vi "RT_Transmission.vi"() -> ()   [LabVIEW 2016]
uses:
  <vilib>/Instr/_visa.llb/VISA Configure Serial Port (Instr).vi
  <vilib>/FPGAPlugInAG/cRIO-9067/niLvFpga_Open_cRIO-9067.vi
  <vilib>/Utility/error.llb/Error Cluster From Error Code.vi
  <vilib>/rvi/errors/niLvFpgaAdjustHostInterfaceError.vi
  <vilib>/functionblocks/Control/PID/PID.vi
  <vilib>/rvi/interface/nirviOpenFPGA/nirviOpenFPGA.xnode
  FPGA Bitfiles/MayUpgrade_FPGA-Trans_Transmission-FPG_MZXtHOBdRVI.lvbitx
  FPGA_Transmission.vi
  <vilib>/rvi/interface/nirviReadWriteControl/nirviReadWriteControl.xnode
  <vilib>/functionblocks/FB Core/FB Core.xnode
  <vilib>/functionblocks/NI_FunctionBlock Libraries.lvlib
  NiFpgaLv.dll
  <vilib>/rvi/errors/niLvFpgaMergeErrorWithErrorCode.vi
panel:
  in  "Tab Control":enum32{"control", "Junk"}(tab)
  out "Steerer X+":dbl
  out "Steerer X-":dbl
  out "Steerer Y+":dbl
  out "Steerer Y-":dbl
  out "ExB +":dbl
  out "ExB -":dbl
  out "X+ V":fxp<+/-,26,5> format="%.23g"
  out "X+ I":fxp<+/-,26,5> format="%_4g"
  out "X- V":fxp<+/-,26,5> format="%_4g"
  out "X-I":fxp<+/-,26,5> format="%_4g"
  out "Y+ V":fxp<+/-,26,5> format="%_4g"
  out "Y+I":fxp<+/-,26,5> format="%_4g"
  out "Y-V":fxp<+/-,26,5> format="%_4g"
  out "Y-I":fxp<+/-,26,5> format="%_4g"
  out "ExB + V":fxp<+/-,26,5> format="%_4g"
  out "ExB +I":fxp<+/-,26,5> format="%_4g"
  out "ExB -V":fxp<+/-,26,5> format="%_4g"
  out "ExB-I":fxp<+/-,26,5> format="%_4g"
  out "ExB Magnet command string":string
  out "Ion gauge switch object cluser 2":T1
  out "Ion gauge anal waist Cluster 1":T1
  out "EXB":dbl
  in  "derivative time (Td, min)":dbl=0.05
  in  "integral time (Ti, min)":dbl=0.01
  in  "proportional gain (Kc)":dbl=25.0
  out "Analyze Magnet command string":string
  out "anal field read":dbl
  out "unsigned byte array":u8[](array[numeric])
  out "Analyze read":u8[](array[numeric])
  out "analyze magnet set field":dbl
  out "element":dbl
  in  "diverter":bool
  out "diverter":bool
  out "ExB Magnet read string":string
  out "ExB Magnet read":dbl
  out "ExB loop error":errorcluster
  out "Analog control error":errorcluster
  out "FPGA error":errorcluster
  in  "Ion gauge cluster control":T1
  out "Convectron 3":u8[](array[numeric])
  out "Ion gauge 4":u8[](array[numeric])
  out "Convectron 4":u8[](array[numeric])
  out "Ion gauge 5":u8[](array[numeric])
  out "Convectron 2":u8[](array[numeric])
  out "Ion gauge 2":u8[](array[numeric])
  out "Convectron 1":u8[](array[numeric])
  out "Ion gauge 1":u8[](array[numeric])
  out "Vac Cluster Error":errorcluster
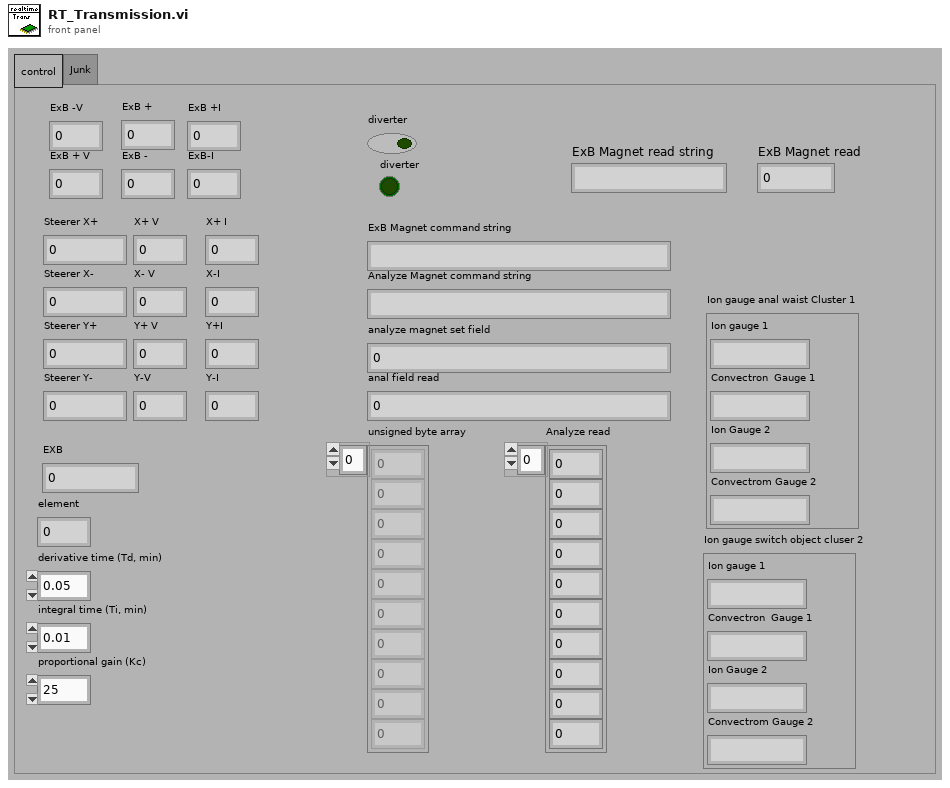
[diagram p1: front panel]
types:
  T1 = cluster{"Ion gauge 1":string, "Convectron  Gauge 1 ":string, "Ion Gauge 2":string, "Convectrom Gauge 2":string}
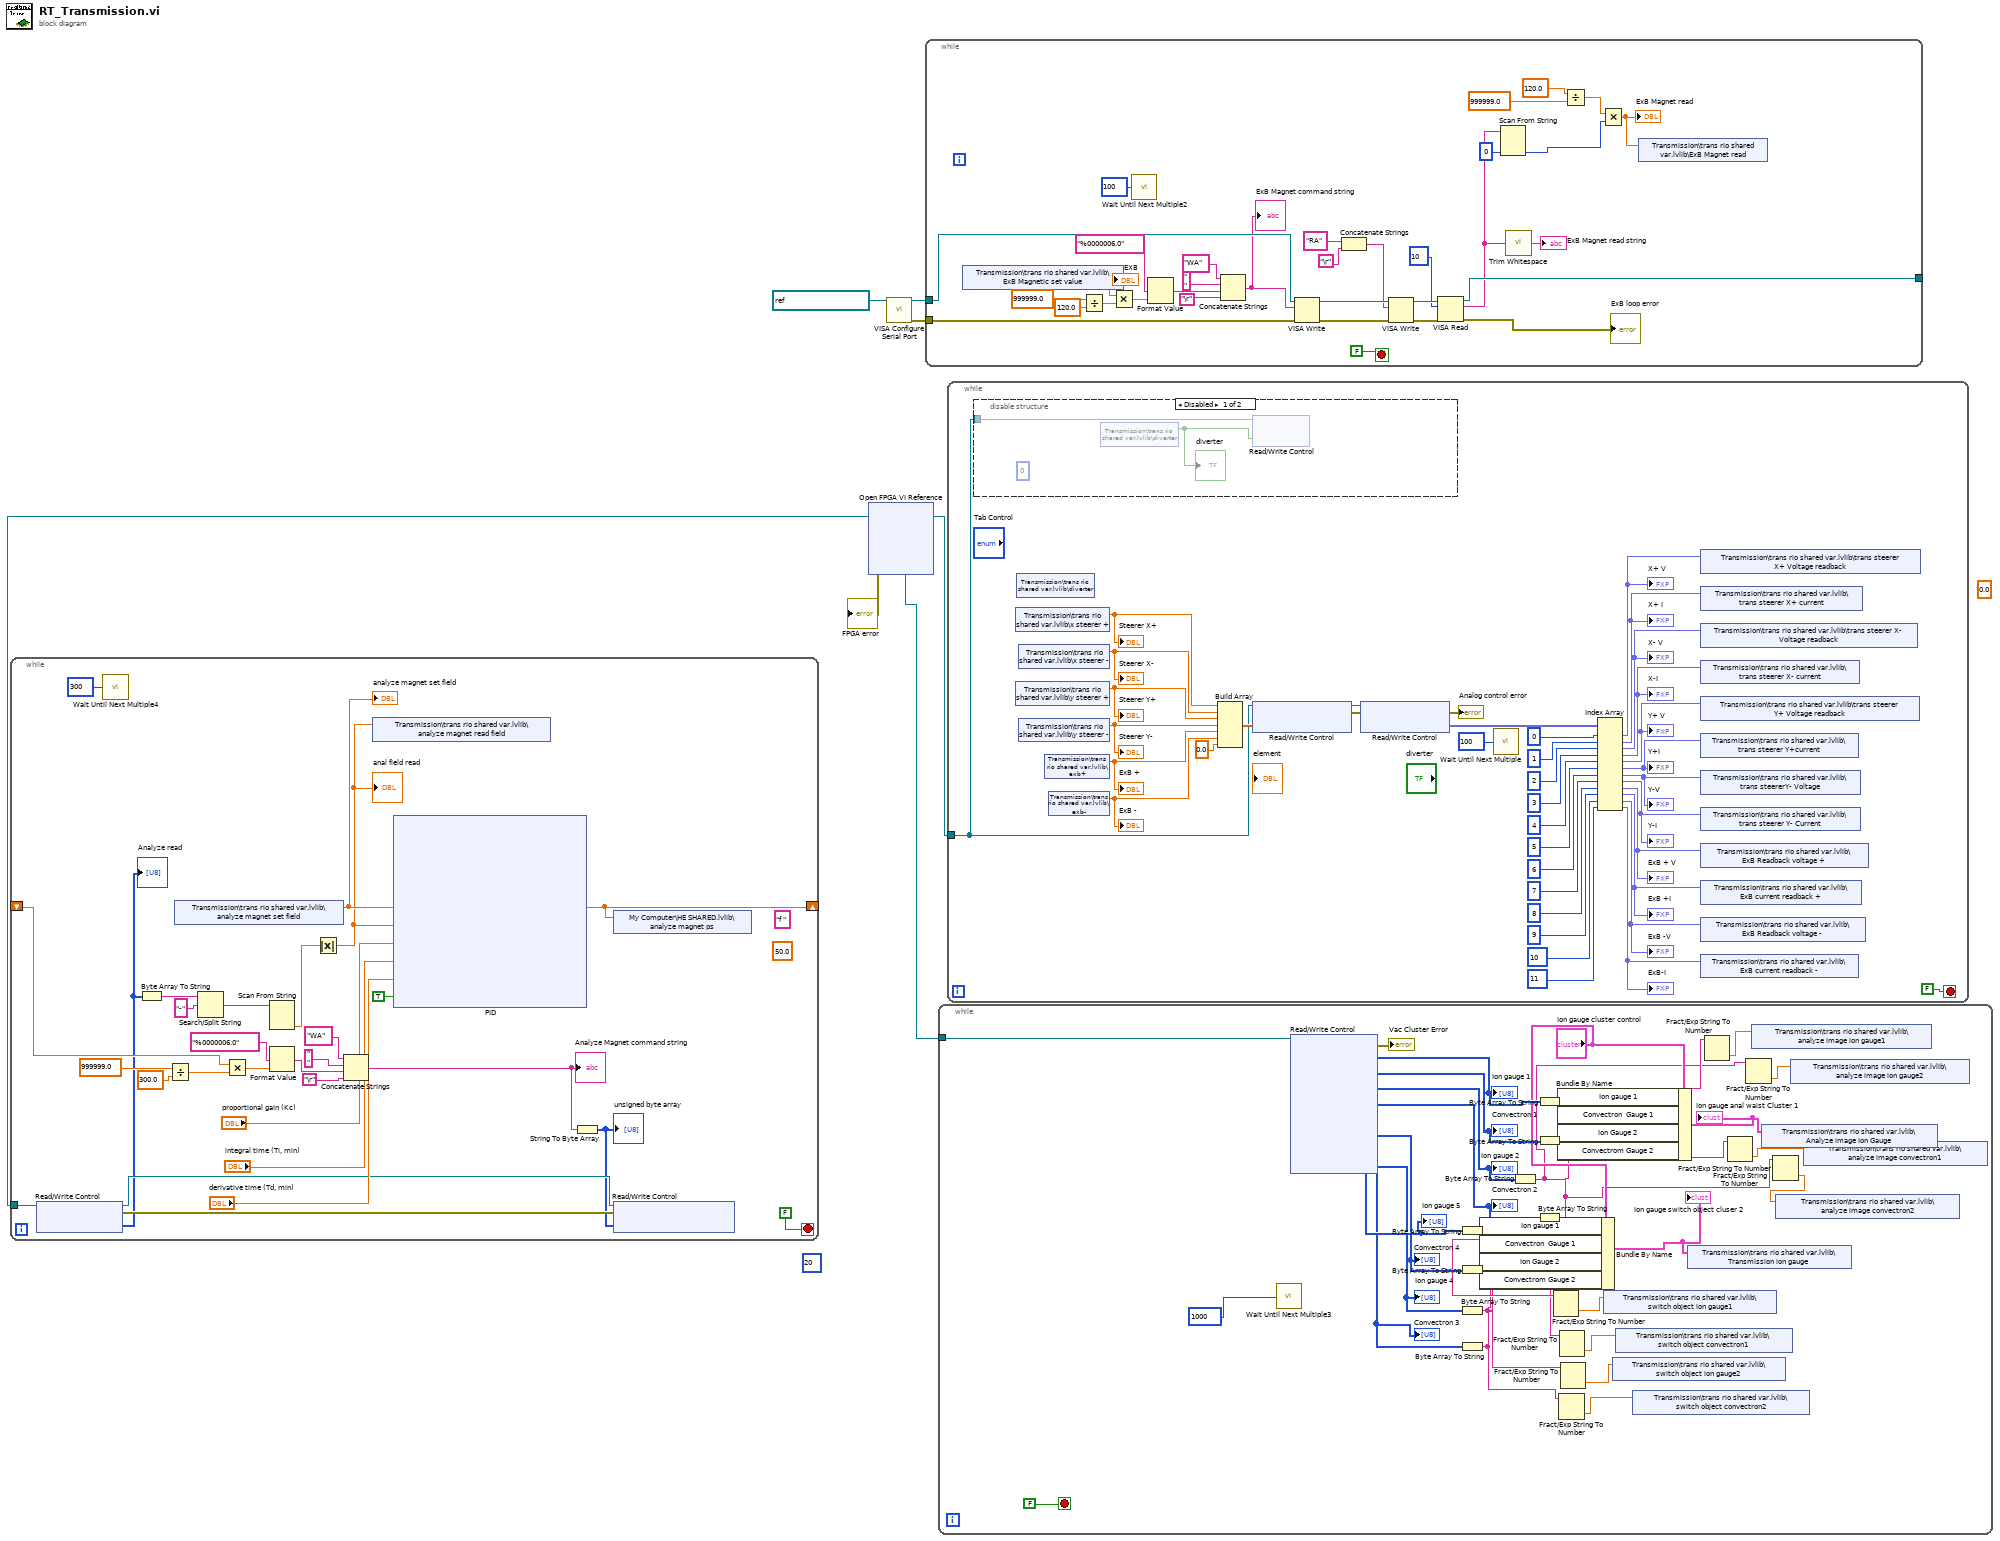
[diagram p0: block diagram]
diagram:
  (unwired) 20 ("dimension size")
  (unwired) 0.0 ("output")
  n1 = xnode "Open FPGA VI Reference"() -> ("FPGA VI Reference Out"=w1:refnum<k20>, "error out"=→"FPGA error":errorcluster)  [unwired: 2 in]
  n2 = while {
    shift-right: [w20] -> _
    shift-left: _ -> [w9]
    tunnel: w1 -> [w14]
    stop <- FALSE stop-if-true
    (unwired) 50.0 ("x")
    (unwired) "f " ("regular expression")
    n3 = xnode "Read/Write Control"("FPGA VI Reference In"=w14) -> ("FPGA VI Reference Out"=w13:refnum<k20>, "error out"=w12:errorcluster, "Analyze read"=w8:u8[])  [unwired: 1 in]
    "Analyze read" <- w8
    n4 = call "Wait Until Next Multiple4"("Count(mSec)"=u32 300 ("millisecond multiple")) -> ()  [unwired: 1 out]
    n5 = Byte Array To String(unsigned byte array=w8) -> (string=w22:string)
    n6 = Divide(x=999999.0, y=300.0) -> (x/y=w27:dbl)
    n7 = shared-variable "Transmission\\trans rio shared var.lvlib\\analyze magnet set field"() -> (w7:dbl)  [unwired: 1 in, 1 out]
    "analyze magnet set field" <- w7
    n8 = Search/Split String(string=w22, search string/char (-)="-") -> (match + rest of string=w10:string)  [unwired: 3 out]
    n9 = Multiply(x=w9, y=w27) -> (x*y=w29:dbl)
    n10 = Scan From String(input string=w10) -> (output 1=w21:dbl)  [unwired: 3 in, 4 out]
    n11 = Format Value(format string="%0000006.0", value (0)=w29) -> (output string=w32:string)  [unwired: 1 out]
    n12 = Absolute Value(x=w21) -> (abs(x)=w6:dbl)
    "anal field read" <- w6
    n13 = Concatenate Strings("WA", " ", w32, "\r") -> (w33:string)
    "Analyze Magnet command string" <- w33
    n14 = shared-variable "Transmission\\trans rio shared var.lvlib\\analyze magnet read field"(w6) -> ()  [unwired: 1 in, 1 out]
    n15 = xnode "PID"("setpoint"=w7, "process variable"=w6, "proportional gain (Kc)"="proportional gain (Kc)", "integral time (Ti, min)"="integral time (Ti, min)", "derivative time (Td, min)"="derivative time (Td, min)", "auto? (T)"=TRUE) -> ("output"=w20:dbl)  [unwired: 1 in, 1 out]
    n16 = String To Byte Array(string=w33) -> (unsigned byte array=w11:u8[])
    "unsigned byte array" <- w11
    n17 = shared-variable "My Computer\\HE SHARED.lvlib\\analyze magnet ps"(w20) -> ()  [unwired: 1 in, 1 out]
    n18 = xnode "Read/Write Control"("FPGA VI Reference In"=w13, "error in"=w12, "analyze ps set array"=w11) -> ()  [unwired: 2 out]
  }
  n19 = call-poly "VISA Configure Serial Port"("VISA resource name"=refnum<visa-resource-name> "ASRL1::INSTR") -> ("VISA resource name out"=w5:refnum<visa-resource-name>, "error out"=w4:errorcluster)  [unwired: 5 in, 8 out]
  n20 = while {
    tunnel: w4 -> [w123]
    tunnel: w5 -> [w122]
    tunnel: [w113] -> _
    stop <- FALSE stop-if-true
    n21 = shared-variable "Transmission\\trans rio shared var.lvlib\\ExB Magnetic set value"() -> (w121:dbl)  [unwired: 1 in, 1 out]
    "EXB" <- w121
    n22 = Divide(x=999999.0, y=120.0) -> (x/y=w131:dbl)
    n23 = Multiply(x=w121, y=w131) -> (x*y=w124:dbl)
    n24 = call "Wait Until Next Multiple2"("Count(mSec)"=u32 100) -> ()  [unwired: 1 out]
    n25 = Format Value(format string="%0000006.0", value (0)=w124) -> (output string=w127:string)  [unwired: 1 out]
    n26 = Concatenate Strings("WA", " ", w127, "\r") -> (w119:string)
    "ExB Magnet command string" <- w119
    n27 = VISA Write(VISA resource name=w122, write buffer=w119, error in (no error)=w123) -> (VISA resource name out=w114:refnum<visa-resource-name>, error out=w117:errorcluster)  [unwired: 1 out]
    n28 = Concatenate Strings("RA" ("write buffer"), "\r" ("string")) -> (w111:string)
    n29 = VISA Write(VISA resource name=w114, write buffer=w111, error in (no error)=w117) -> (VISA resource name out=w115:refnum<visa-resource-name>, error out=w118:errorcluster)  [unwired: 1 out]
    n30 = VISA Read(VISA resource name=w115, byte count=u32 10, error in (no error)=w118) -> (VISA resource name out=w113:refnum<visa-resource-name>, read buffer=w103:string, error out=→"ExB loop error":errorcluster)  [unwired: 1 out]
    n31 = Scan From String(input string=w103, default 1=u32 0 ("default value 1")) -> (output 1=w104:u32)  [unwired: 3 in, 3 out]
    n32 = call <vilib>:"Trim Whitespace.vi"("string"=w103) -> ("trimmed string"=→"ExB Magnet read string":string)  [unwired: 1 in]
    n33 = Divide(x=120.0 ("y"), y=999999.0 ("x")) -> (x/y=w105:dbl)
    n34 = Multiply(x=w105, y=w104) -> (x*y=w101:dbl)
    "ExB Magnet read" <- w101
    n35 = shared-variable "Transmission\\trans rio shared var.lvlib\\ExB Magnet read"(w101) -> ()  [unwired: 1 in, 1 out]
  }
  n36 = while {
    tunnel: w1 -> [w152]
    stop <- FALSE stop-if-true
    n37 = call "Wait Until Next Multiple3"("Count(mSec)"=u32 1000 ("millisecond multiple")) -> ()  [unwired: 1 out]
    n38 = xnode "Read/Write Control"("FPGA VI Reference In"=w152) -> ("error out"=→"Vac Cluster Error":errorcluster, "Ion gauge 1"=w161:u8[], "Convectron 1"=w162:u8[], "Ion gauge 2"=w163:u8[], "Convectron 2"=w164:u8[], "Ion gauge 3"=w158:u8[], "Convectron 3"=w157:u8[], "Convectron 4"=w155:u8[], "Ion gauge 4"=w156:u8[])  [unwired: 1 in, 1 out]
    "Ion gauge 1" <- w161
    "Convectron 1" <- w162
    "Ion gauge 2" <- w163
    "Convectron 2" <- w164
    "Ion gauge 5" <- w158
    "Convectron 4" <- w157
    "Ion gauge 4" <- w156
    "Convectron 3" <- w155
    n39 = Byte Array To String(unsigned byte array=w158) -> (string=w149:string)
    n40 = Byte Array To String(unsigned byte array=w157) -> (string=w148:string)
    n41 = Byte Array To String(unsigned byte array=w156) -> (string=w147:string)
    n42 = Byte Array To String(unsigned byte array=w155) -> (string=w146:string)
    n43 = Bundle By Name(cluster="Ion gauge cluster control", "Ion gauge 1"=w149, "Convectron  Gauge 1"=w148, "Ion Gauge 2"=w147, "Convectrom Gauge 2"=w146) -> (w151:T1)
    "Ion gauge switch object cluser 2" <- w151
    n44 = Byte Array To String(unsigned byte array=w163) -> (string=w138:string)
    n45 = Byte Array To String(unsigned byte array=w161) -> (string=w141:string)
    n46 = Byte Array To String(unsigned byte array=w162) -> (string=w140:string)
    n47 = Byte Array To String(unsigned byte array=w164) -> (string=w139:string)
    n48 = Fract/Exp String To Number(string=w149) -> (number=w145:dbl)  [unwired: 3 in, 1 out]
    n49 = Bundle By Name(cluster="Ion gauge cluster control", "Ion gauge 1"=w141, "Convectron  Gauge 1"=w140, "Ion Gauge 2"=w138, "Convectrom Gauge 2"=w139) -> (w150:T1)
    "Ion gauge anal waist Cluster 1" <- w150
    n50 = Fract/Exp String To Number(string=w146) -> (number=w142:dbl)  [unwired: 3 in, 1 out]
    n51 = Fract/Exp String To Number(string=w148) -> (number=w144:dbl)  [unwired: 3 in, 1 out]
    n52 = Fract/Exp String To Number(string=w147) -> (number=w143:dbl)  [unwired: 3 in, 1 out]
    n53 = shared-variable "Transmission\\trans rio shared var.lvlib\\switch object ion gauge1"(w145) -> ()  [unwired: 1 in, 1 out]
    n54 = shared-variable "Transmission\\trans rio shared var.lvlib\\switch object ion gauge2"(w143) -> ()  [unwired: 1 in, 1 out]
    n55 = shared-variable "Transmission\\trans rio shared var.lvlib\\switch object convectron1"(w144) -> ()  [unwired: 1 in, 1 out]
    n56 = shared-variable "Transmission\\trans rio shared var.lvlib\\switch object convectron2"(w142) -> ()  [unwired: 1 in, 1 out]
    n57 = shared-variable "Transmission\\trans rio shared var.lvlib\\Transmission ion gauge"(w151) -> ()  [unwired: 1 in, 1 out]
    n58 = Fract/Exp String To Number(string=w141) -> (number=w137:dbl)  [unwired: 3 in, 1 out]
    n59 = Fract/Exp String To Number(string=w140) -> (number=w135:dbl)  [unwired: 3 in, 1 out]
    n60 = Fract/Exp String To Number(string=w138) -> (number=w136:dbl)  [unwired: 3 in, 1 out]
    n61 = shared-variable "Transmission\\trans rio shared var.lvlib\\analyze image ion gauge1"(w137) -> ()  [unwired: 1 in, 1 out]
    n62 = shared-variable "Transmission\\trans rio shared var.lvlib\\Analyze image Ion Gauge"(w150) -> ()  [unwired: 1 in, 1 out]
    n63 = Fract/Exp String To Number(string=w139) -> (number=w134:dbl)  [unwired: 3 in, 1 out]
    n64 = shared-variable "Transmission\\trans rio shared var.lvlib\\analyze image convectron2"(w134) -> ()  [unwired: 1 in, 1 out]
    n65 = shared-variable "Transmission\\trans rio shared var.lvlib\\analyze image ion gauge2"(w136) -> ()  [unwired: 1 in, 1 out]
    n66 = shared-variable "Transmission\\trans rio shared var.lvlib\\analyze image convectron1"(w135) -> ()  [unwired: 1 in, 1 out]
  }
  n67 = while {
    tunnel: w1 -> [w165]
    stop <- FALSE stop-if-true
    n68 = disable-structure shown="Disabled" {
      disable-tunnel: w165 -> [w205 _]
      frame Disabled {
        (unwired) 0 ("dimension size")
        n69 = shared-variable "Transmission\\trans rio shared var.lvlib\\diverter"() -> (w204:bool)  [unwired: 1 in, 1 out]
        "diverter" <- w204
        n70 = xnode "Read/Write Control"("FPGA VI Reference In"=w205, "diverter"=w204) -> ()  [unwired: 1 in, 2 out]
      }
      frame Enabled {
      }
    }
    n71 = shared-variable "Transmission\\trans rio shared var.lvlib\\x steerer +"() -> (w184:dbl)  [unwired: 1 in, 1 out]
    "Steerer X+" <- w184
    n72 = shared-variable "Transmission\\trans rio shared var.lvlib\\y steerer +"() -> (w186:dbl)  [unwired: 1 in, 1 out]
    "Steerer Y+" <- w186
    n73 = shared-variable "Transmission\\trans rio shared var.lvlib\\diverter"() -> ()  [unwired: 1 in, 2 out]
    n74 = shared-variable "Transmission\\trans rio shared var.lvlib\\x steerer -"() -> (w185:dbl)  [unwired: 1 in, 1 out]
    "Steerer X-" <- w185
    n75 = shared-variable "Transmission\\trans rio shared var.lvlib\\y steerer -"() -> (w187:dbl)  [unwired: 1 in, 1 out]
    "Steerer Y-" <- w187
    n76 = shared-variable "Transmission\\trans rio shared var.lvlib\\exb+"() -> (w188:dbl)  [unwired: 1 in, 1 out]
    "ExB +" <- w188
    n77 = shared-variable "Transmission\\trans rio shared var.lvlib\\exb-"() -> (w189:dbl)  [unwired: 1 in, 1 out]
    "ExB -" <- w189
    n78 = Build Array(w184, w185, w186, w187, w188, w189, 0.0 ("element")) -> (w203:dbl[])
    n79 = xnode "Read/Write Control"("FPGA VI Reference In"=w165, "Analog Output"=w203) -> ("FPGA VI Reference Out"=w169:refnum<k20>, "error out"=w168:errorcluster)  [unwired: 1 in]
    n80 = xnode "Read/Write Control"("FPGA VI Reference In"=w169, "error in"=w168) -> ("error out"=→"Analog control error":errorcluster, "Analog input"=w170:fxp<+/-,26,5>[])  [unwired: 1 out]
    n81 = call "Wait Until Next Multiple"("Count(mSec)"=u32 100) -> ()  [unwired: 1 out]
    n82 = Index Array(array=w170, index #1=0 ("index"), index #2=1 ("index"), index #3=2 ("index"), index #4=3 ("index"), index #5=4 ("index"), index #6=5 ("index"), index #7=6 ("index"), index #8=7 ("index"), index #9=8 ("index"), index #10=9 ("index"), index #11=10 ("index"), index #12=11 ("index")) -> (element #1=w182:fxp<+/-,26,5>, element #2=w180:fxp<+/-,26,5>, element #3=w181:fxp<+/-,26,5>, element #4=w183:fxp<+/-,26,5>, element #5=w179:fxp<+/-,26,5>, element #6=w177:fxp<+/-,26,5>, element #7=w178:fxp<+/-,26,5>, element #8=w176:fxp<+/-,26,5>, element #9=w175:fxp<+/-,26,5>, element #10=w173:fxp<+/-,26,5>, element #11=w174:fxp<+/-,26,5>, element #12=w172:fxp<+/-,26,5>)
    "X+ V" <- w182
    "X+ I" <- w180
    "X- V" <- w181
    "X-I" <- w183
    "Y+ V" <- w179
    "Y+I" <- w177
    "Y-V" <- w178
    "Y-I" <- w176
    "ExB + V" <- w175
    "ExB +I" <- w173
    "ExB -V" <- w174
    "ExB-I" <- w172
    n83 = shared-variable "Transmission\\trans rio shared var.lvlib\\trans steerer X+ Voltage readback"(w182) -> ()  [unwired: 1 in, 1 out]
    n84 = shared-variable "Transmission\\trans rio shared var.lvlib\\trans steerer X+ current"(w180) -> ()  [unwired: 1 in, 1 out]
    n85 = shared-variable "Transmission\\trans rio shared var.lvlib\\trans steerer X- Voltage readback"(w181) -> ()  [unwired: 1 in, 1 out]
    n86 = shared-variable "Transmission\\trans rio shared var.lvlib\\trans steerer X- current"(w183) -> ()  [unwired: 1 in, 1 out]
    n87 = shared-variable "Transmission\\trans rio shared var.lvlib\\trans steerer Y+ Voltage readback"(w179) -> ()  [unwired: 1 in, 1 out]
    n88 = shared-variable "Transmission\\trans rio shared var.lvlib\\trans steerer Y+current"(w177) -> ()  [unwired: 1 in, 1 out]
    n89 = shared-variable "Transmission\\trans rio shared var.lvlib\\trans steererY- Voltage"(w178) -> ()  [unwired: 1 in, 1 out]
    n90 = shared-variable "Transmission\\trans rio shared var.lvlib\\trans steerer Y- Current"(w176) -> ()  [unwired: 1 in, 1 out]
    n91 = shared-variable "Transmission\\trans rio shared var.lvlib\\ExB Readback voltage +"(w175) -> ()  [unwired: 1 in, 1 out]
    n92 = shared-variable "Transmission\\trans rio shared var.lvlib\\ExB current readback +"(w173) -> ()  [unwired: 1 in, 1 out]
    n93 = shared-variable "Transmission\\trans rio shared var.lvlib\\ExB Readback voltage -"(w174) -> ()  [unwired: 1 in, 1 out]
    n94 = shared-variable "Transmission\\trans rio shared var.lvlib\\ExB current readback -"(w172) -> ()  [unwired: 1 in, 1 out]
  }
